vi "FGV UE Tiempo.vi"(11 "Enum":T1) -> (3 "User Event out":refnum<user-event>)   [LabVIEW 2020]
uses:
  Options.ctl
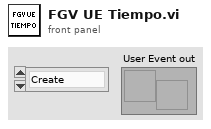
[diagram p1: front panel]
types:
  T1 = typedef "Options.ctl" = enum16{"Create", "Get", "Destroy"}
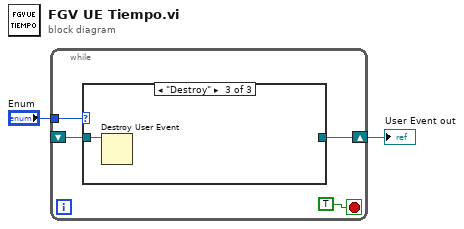
[diagram p0: block diagram]
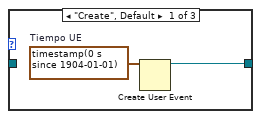
[diagram p2: hidden frame]
diagram:
  n1 = while {
    tunnel: "Enum" -> [w6]
    shift-right: [w5] -> w1
    shift-left: _ -> [w3]
    stop <- TRUE stop-if-true
    n2 = case shown="\"Destroy\"" w6 {
      tunnel: [w8 w9 _] -> w5
      tunnel: w3 -> [_ w9 w10]
      frame "Create", Default {
        w7 = timestamp(0 s since 1904-01-01)  # Tiempo UE
        n3 = Create User Event(user event datatype=w7) -> (user event=w8:refnum<user-event>)  [unwired: 1 in, 1 out]
      }
      frame "Get" {
      }
      frame "Destroy" {
        n4 = Destroy User Event(user event=w10) -> ()  [unwired: 1 in, 1 out]
      }
    }
  }
  "User Event out" <- w1
